vi "GetStrArrTo2DimenArrayCtrl.vi"(11 "array in":refnum<vi>) -> (2 "arr data":string[][](array[string]), 3 "array out":refnum<vi>)   [LabVIEW 2018, in "Library-Ctrl.lvlib"]
uses:
  Library-Ctrl.lvlib
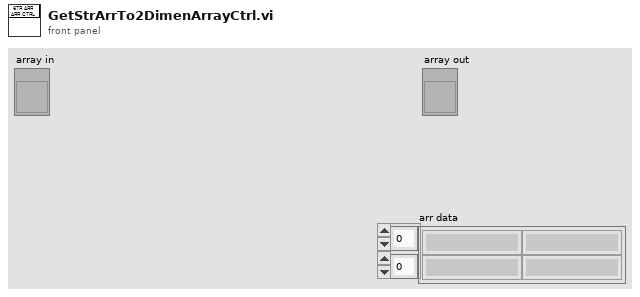
[diagram p1: front panel]
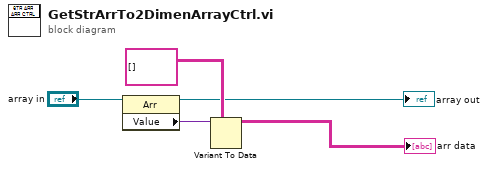
[diagram p0: block diagram]
diagram:
  n1 = property class="Arr"(reference="array in") -> (reference out=→"array out":refnum<vi>, "Value"=w4:variant)  [unwired: 1 in, 1 out]
  n2 = Variant To Data(type=string[][] [] ("array data"), Variant=w4) -> (data=→"arr data":string[][])  [unwired: 1 in, 1 out]
